vi "Set Label Prepend Append.vi"(5 "Label Append":string, 7 "Label Prepend":string, 8 "error in (no error)":errorcluster, 11 "CConfig Variant Accessor in":refnum<class "CConfig Variant Accessor.lvclass">) -> (0 "error out":errorcluster, 3 "CConfig Variant Accessor out":refnum<class "CConfig Variant Accessor.lvclass">)   [LabVIEW 2013, in "CConfig Variant Accessor.lvclass"]
doc: "Copyright 2018, Carya Automatisering, Wiebe Walstra."
uses:
  CConfig Variant Accessor.lvclass
  CConfig Variant Accessor.lvclass/CConfig Variant Accessor.ctl
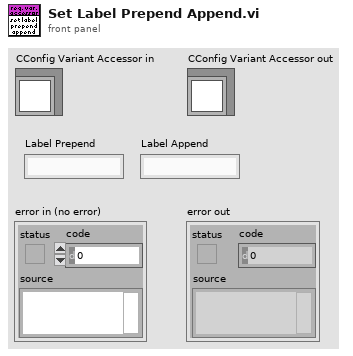
[diagram p1: front panel]
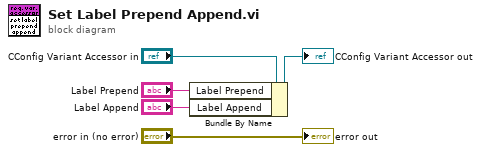
[diagram p0: block diagram]
diagram:
  n1 = Bundle By Name(cluster="CConfig Variant Accessor in", "Label Prepend"="Label Prepend", "Label Append"="Label Append") -> (→"CConfig Variant Accessor out":refnum<class "CConfig Variant Accessor.lvclass">)
  "error out" <- "error in (no error)"
